vi "XY_coordinate.vi"() -> (3 "XY_Coordinate":picture)   [LabVIEW 2011]
panel:
  out "strInfo":string
  out "Pic_Right":u32
  out "Pic_Left":i32
  out "mu08ObjectNum":u8
  out "ms16EachXYHigh":i16
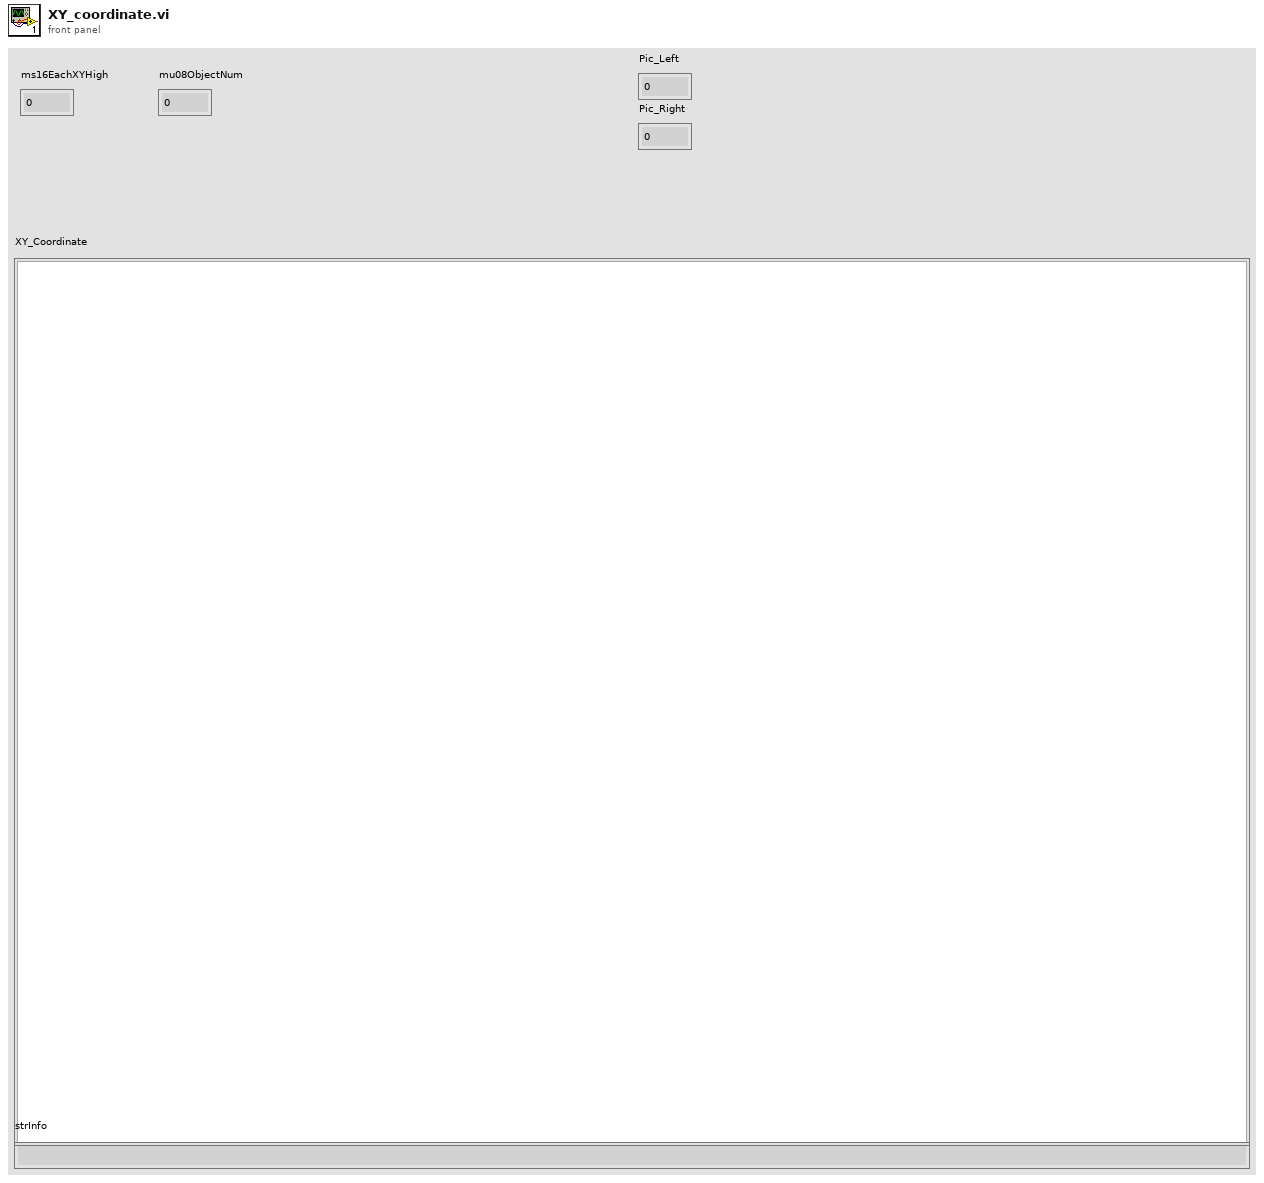
[diagram p1: front panel]
types:
  T1 = cluster{"Width":u16, "Style":enum32{"Solid", "Dash", "Dot", "DashDot", "DashDotDot"}}
  T2 = typedef "LVBoundsTypeDef.ctl" = cluster{"Width":u32, "Height":u32}
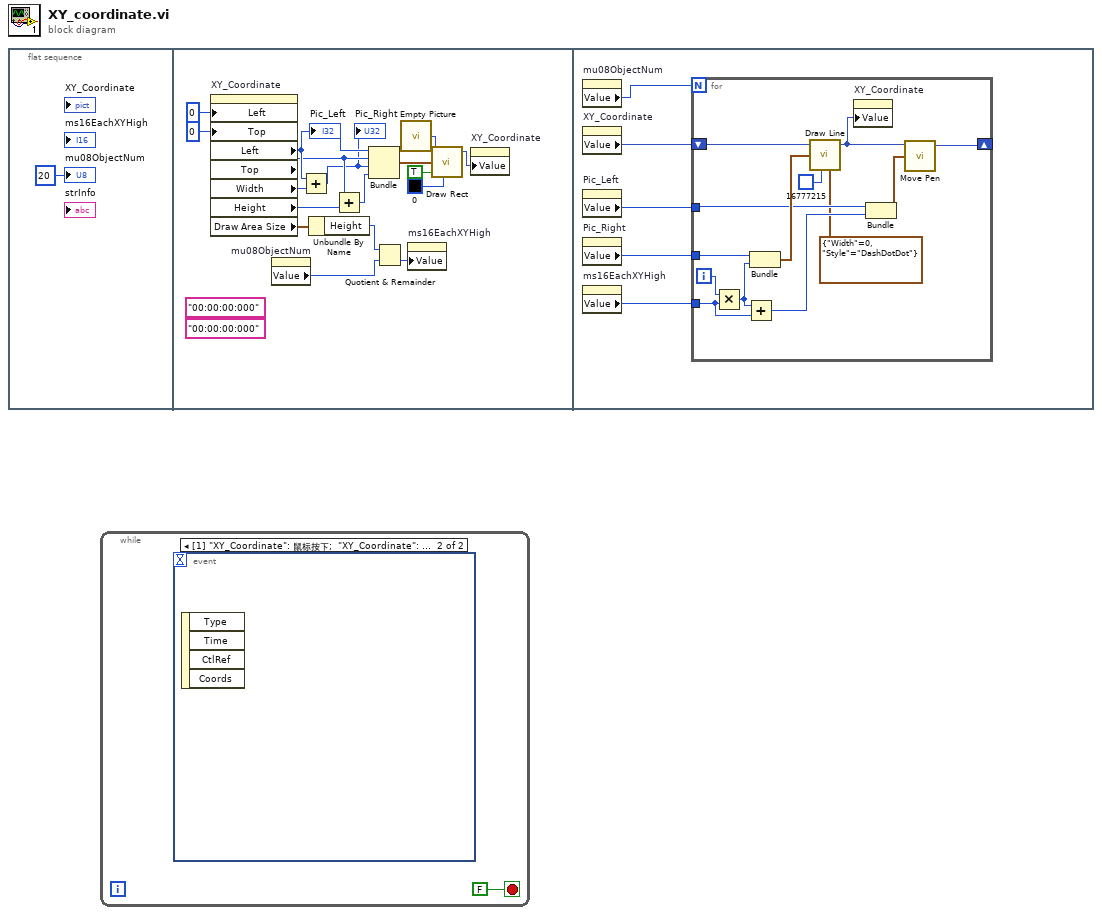
[diagram p0: block diagram]
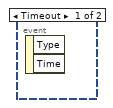
[diagram p2: hidden frame]
diagram:
  n1 = flat-sequence {
    frame #0 {
      "mu08ObjectNum" <- u8 20 ("mu08ObjectNum")
    }
    frame #1 {
      (unwired) "00:00:00:000"
      (unwired) "00:00:00:000"
      n2 = property on="XY_Coordinate" class="Pict"("Left"=0 ("位置:居左"), "Top"=0 ("位置:置顶")) -> ("Left"=w15:i32, "Top"=w12:i32, "Width"=w14:u32, "Height"=w13:u32, "Draw Area Size"=w6:T2)  [unwired: 2 in, 2 out]
      "Pic_Left" <- w15
      n3 = property on="mu08ObjectNum" class="DigNum (严格)"() -> ("Value"=w4:u8)  [unwired: 2 in, 2 out]
      n4 = Add(x=w15, y=w14) -> (x+y=w2:u32)
      "Pic_Right" <- w2
      n5 = Unbundle By Name(w6) -> ("Height"=w5:u32)
      n6 = Add(x=w12, y=w13) -> (x+y=w11:u32)
      n7 = Bundle("Left"=w15, "Top"=w12, w2, w11) -> (w10:cluster{"Left":i32, "Top":i32, u32, u32})  [unwired: 1 in]
      n8 = Quotient & Remainder(x=w5, y=w4) -> (floor(x/y)=w3:u32)  [unwired: 1 out]
      n9 = call "Empty Picture"() -> ("empty picture"=w16:picture)
      n10 = property on="ms16EachXYHigh" class="DigNum (严格)"("Value"=w3) -> ()  [unwired: 2 in, 2 out]
      n11 = call <vilib>:"Draw Rect.vi"("picture"=w16, "rect"=w10, "fill?(F)"=TRUE, "color(black)"=u32 0) -> ("new picture"=w7:picture)  [unwired: 5 in]
      n12 = property on="XY_Coordinate" class="Pict"("Value"=w7) -> ()  [unwired: 2 in, 2 out]
    }
    frame #2 {
      n13 = property on="mu08ObjectNum" class="DigNum (严格)"() -> ("Value"=w23:u8)  [unwired: 2 in, 2 out]
      n14 = property on="XY_Coordinate" class="Pict"() -> ("Value"=w22:picture)  [unwired: 2 in, 2 out]
      n15 = property on="Pic_Left" class="DigNum (严格)"() -> ("Value"=w21:i32)  [unwired: 2 in, 2 out]
      n16 = property on="Pic_Right" class="DigNum (严格)"() -> ("Value"=w20:u32)  [unwired: 2 in, 2 out]
      n17 = property on="ms16EachXYHigh" class="DigNum (严格)"() -> ("Value"=w19:i16)  [unwired: 2 in, 2 out]
      n18 = for {
        N: w23 -> [_]
        shift-right: [w30] -> _
        shift-left: w22 -> [w36]
        tunnel: w21 -> [w29]
        tunnel: w20 -> [w34]
        tunnel: w19 -> [w26]
        i -> [w35]
        n19 = Multiply(x=w35, y=w26) -> (x*y=w27:i32)
        n20 = Add(x=w27, y=w26) -> (x+y=w25:i32)
        n21 = Bundle("Value"=w34, w27) -> (w33:cluster{"Value":u32, i32})  [unwired: 1 in]
        n22 = call <vilib>:"Draw Line.vi"("picture"=w36, "end point"=w33, "color(black)"=u32 16777215, "pen"=T1 {"Width"=0, "Style"=enum."DashDotDot"}) -> ("new picture"=w31:picture)  [unwired: 5 in]
        n23 = property on="XY_Coordinate" class="Pict"("Value"=w31) -> ()  [unwired: 2 in, 2 out]
        n24 = Bundle("Value"=w29, w25) -> (w28:cluster{"Value":i32, i32})  [unwired: 1 in]
        n25 = call <vilib>:"Move Pen.vi"("new position"=w28, "picture"=w31) -> ("new picture"=w30:picture)  [unwired: 3 in]
      }
    }
  }
  n26 = while {
    stop <- FALSE stop-if-true
    n27 = event shown="[1] \"XY_Coordinate\": 鼠标按下;  \"XY_Coordinate\": 鼠标移动" {
      selector: _ -> [_ _]
      dyn-events: _ -> [_ _]
      timeout: _ -> [_ _]
      event Timeout {
        n28 = event-data() -> ()  [unwired: 1 in, 2 out]
      }
      event "XY_Coordinate": Mouse Down; "XY_Coordinate": Mouse Move {
        n29 = event-data() -> ()  [unwired: 1 in, 4 out]
      }
    }
  }
